vi "Parse HTML.vi"(8 "error in":errorcluster, 11 "result string in":string) -> (0 "error out":errorcluster, 1 "data":string, 3 "result string out":string)   [LabVIEW 2018]
panel:
  out "offset of match":i32
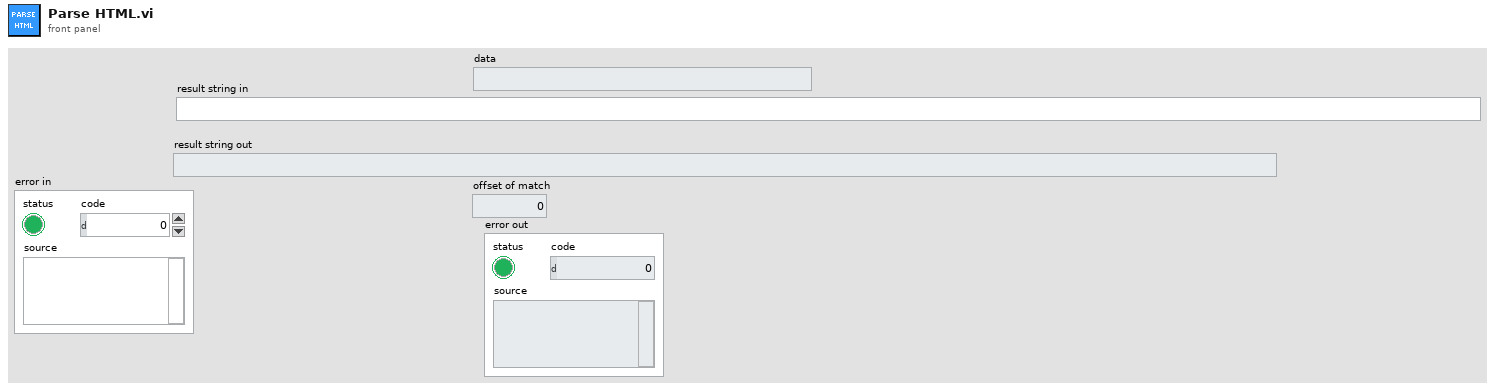
[diagram p1: front panel]
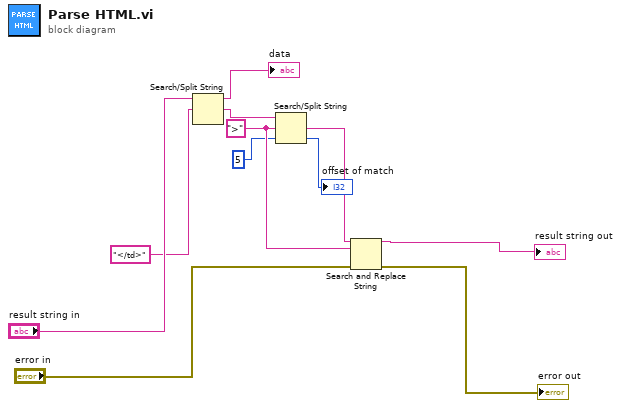
[diagram p0: block diagram]
diagram:
  w6 = ">" ("search string/char (-)")
  n1 = Search/Split String(string="result string in", search string/char (-)="</td>") -> (substring before match=→"data":string, match + rest of string=w7:string)  [unwired: 1 in, 1 out]
  n2 = Search/Split String(string=w7, search string/char (-)=w6, offset (0)=5) -> (match + rest of string=w5:string, offset of match=→"offset of match":i32)  [unwired: 1 out]
  n3 = Search and Replace String(input string=w5, search string=w6, error in="error in") -> (result string=→"result string out":string, error out=→"error out":errorcluster)  [unwired: 5 in, 2 out]
